vi "Drive Encoders Activate.vi"(11 "Encoder Reset":bool) -> (2 "Distance":dbl)   [LabVIEW 2012]
uses:
  <vilib>/Rock Robotics/WPI/DriverStation/DriverStationLCD/WPI_DriverStationLCDLCDLine.ctl
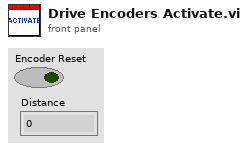
[diagram p1: front panel]
types:
  T1 = typedef "WPI_DriverStationLCDLCDLine.ctl" = enum16{"Main - Line 1", "User - Line 2", "User - Line 3", "User - Line 4", "User - Line 5", "User - Line 6"}
  T2 = typedef "WPI_EncoderDevRef.ctl" = cluster{"DevStatus":errorcluster, "EncoderIndex":T3, "CounterIndex":T4, "DistancePerCount":dbl, "Decoding Type":T5}
  T3 = typedef "FPGA_EncoderIdx.ctl" = enum8{"Enc 0", "Enc 1", "Enc 2", "Enc 3", "Invalid"}
  T4 = typedef "FPGA_CounterCtrSystemIndex.ctl" = enum8{"Ctr 0", "Ctr 1", "Ctr 2", "Ctr 3", "Ctr 4", "Ctr 5", "Ctr 6", "Ctr 7", "Invalid"}
  T5 = typedef "WPI_EncoderType.ctl" = enum16{"1x", "2x", "4x"}
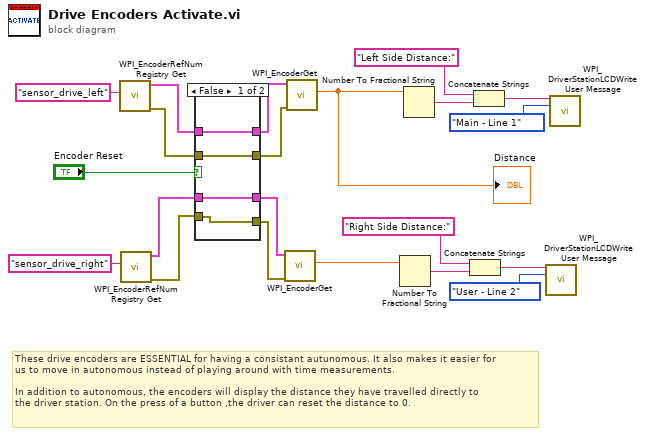
[diagram p0: block diagram]
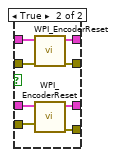
[diagram p2: hidden frame]
diagram:
  # "These drive encoders are ESSENTIAL for having a consistant autunomous. It also makes it easier for \nus to move in autonomous instead of playing around with time measurements. \n\nIn addition to autonomous, the encoders will display the distance they have travelled directly to \nthe driver station. On the press of a button ,the driver can reset the distance to 0."
  n1 = call <vilib>:"WPI_EncoderRefNum Registry Get.vi"("refnum name"="sensor_drive_left") -> ("error out"=w9:errorcluster, "EncoderDevRef"=w10:T2)  [unwired: 9 in]
  n2 = call <vilib>:"WPI_EncoderRefNum Registry Get.vi"("refnum name"="sensor_drive_right") -> ("error out"=w5:errorcluster, "EncoderDevRef"=w6:T2)  [unwired: 9 in]
  n3 = case shown="False" "Encoder Reset" {
    tunnel: w10 -> [w25 w33]
    tunnel: w9 -> [w24 w32]
    tunnel: [w25 w31] -> w8
    tunnel: [w24 w30] -> w7
    tunnel: w6 -> [w23 w29]
    tunnel: w5 -> [w22 w28]
    tunnel: [w23 w27] -> w4
    tunnel: [w22 w26] -> w3
    frame False {
    }
    frame True {
      n4 = call <vilib>:"WPI_EncoderReset.vi"("error in (no error)"=w32, "EncoderDevRef"=w33) -> ("error out"=w30:errorcluster, "EncoderDevRef"=w31:T2)  [unwired: 8 in]
      n5 = call <vilib>:"WPI_EncoderReset.vi"("error in (no error)"=w28, "EncoderDevRef"=w29) -> ("error out"=w26:errorcluster, "EncoderDevRef"=w27:T2)  [unwired: 8 in]
    }
  }
  n6 = call <vilib>:"WPI_EncoderGet.vi"("error in (no error)"=w3, "EncoderDevRef"=w4) -> ("Distance"=w2:dbl)  [unwired: 4 in, 5 out]
  n7 = call <vilib>:"WPI_EncoderGet.vi"("error in (no error)"=w7, "EncoderDevRef"=w8) -> ("Distance"=w1:dbl)  [unwired: 4 in, 5 out]
  "Distance" <- w1
  n8 = Number To Fractional String(number=w2) -> (F-format string=w12:string)  [unwired: 3 in]
  n9 = Number To Fractional String(number=w1) -> (F-format string=w19:string)  [unwired: 3 in]
  n10 = Concatenate Strings("Right Side Distance:" ("string"), w12) -> (w14:string)
  n11 = Concatenate Strings("Left Side Distance:" ("string"), w19) -> (w17:string)
  n12 = call <vilib>:"WPI_DriverStationLCDWrite User Message.vi"("line text"=w14, "line"=WPI_DriverStationLCDLCDLine."User - Line 2") -> ()  [unwired: 13 in, 1 out]
  n13 = call <vilib>:"WPI_DriverStationLCDWrite User Message.vi"("line text"=w17, "line"=WPI_DriverStationLCDLCDLine."Main - Line 1") -> ()  [unwired: 13 in, 1 out]
